vi "TEST Object Manual Bounds (Splitter).vi"() -> ()   [LabVIEW 2021, in "IObject.lvclass"]
uses:
  IObject.lvclass
  <vilib>/Utility/miscctls.llb/LVRectTypeDef.ctl
  Object/Object.lvclass
  C:/Projects/Dynamic-Scaling/Dynamic Scaling/IObject.lvclass
  IContainer/Viewport/Viewport.lvclass
  IContainer/Divider/Divider.lvclass
panel:
  in  "Vertical? [F, hor.]":bool=TRUE
  in  "OK Button 4":bool
  in  "OK Button 3":dbl(graph)
  in  "OK Button 2":dbl(graph)
  in  "Bounds":T1={"Left"=200, "Top"=20, "Right"=550, "Bottom"=190}
  in  "OK Button 1":bool
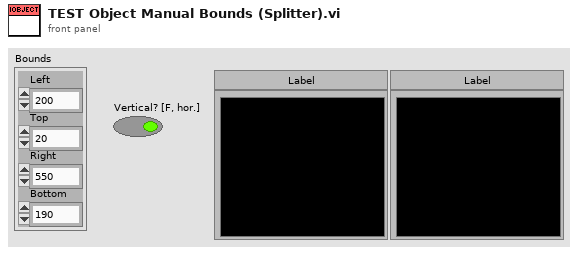
[diagram p1: front panel]
types:
  T1 = typedef "LVRectTypeDef.ctl" = cluster{"Left":i16, "Top":i16, "Right":i16, "Bottom":i16}
  T2 = cluster{"Left":dbl, "Top":dbl, "Right":dbl, "Bottom":dbl}[]
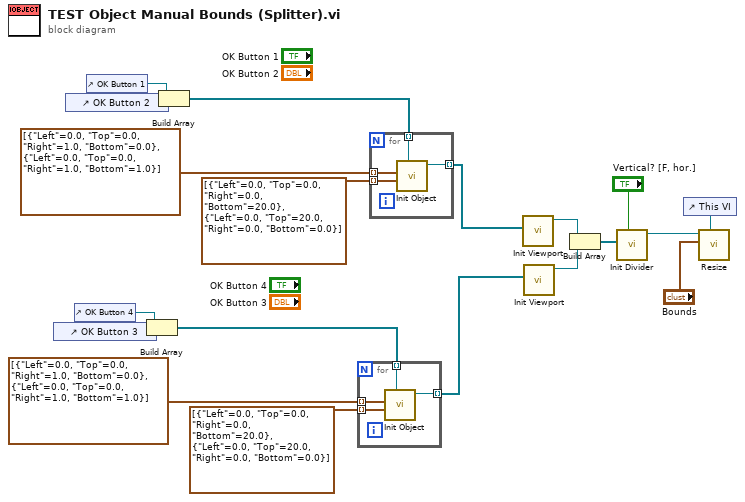
[diagram p0: block diagram]
diagram:
  n1 = control-ref of="OK Button 3"() -> (w7:refnum<vi>)
  n2 = control-ref of="OK Button 2"() -> (w18:refnum<vi>)
  n3 = control-ref of="OK Button 4"() -> (w6:refnum<vi>)
  n4 = control-ref of="OK Button 1"() -> (w19:refnum<vi>)
  n5 = Build Array(w6, w7) -> (w8:refnum<vi>[])
  n6 = Build Array(w19, w18) -> (w17:refnum<vi>[])
  n7 = for {
    tunnel: T2 [{"Left"=0.0, "Top"=0.0, "Right"=1.0, "Bottom"=0.0}, {"Left"=0.0, "Top"=0.0, "Right"=1.0, "Bottom"=1.0}] -> [w23] mode=indexing
    tunnel: w8 -> [w22] mode=indexing
    tunnel: T2 [{"Left"=0.0, "Top"=0.0, "Right"=0.0, "Bottom"=20.0}, {"Left"=0.0, "Top"=20.0, "Right"=0.0, "Bottom"=0.0}] -> [w21] mode=indexing
    tunnel: [w20] -> w11 mode=indexing
    n8 = call "Init Object.vi"("GObj Refnum"=w22, "B [0, 0, 0, 0]"=w21, "A [0, 0, 1, 1]"=w23) -> ("MMI Scaling out"=w20:refnum<class "Object.lvclass">)  [unwired: 7 in, 1 out]
  }
  n9 = for {
    tunnel: T2 [{"Left"=0.0, "Top"=0.0, "Right"=1.0, "Bottom"=0.0}, {"Left"=0.0, "Top"=0.0, "Right"=1.0, "Bottom"=1.0}] -> [w27] mode=indexing
    tunnel: w17 -> [w26] mode=indexing
    tunnel: T2 [{"Left"=0.0, "Top"=0.0, "Right"=0.0, "Bottom"=20.0}, {"Left"=0.0, "Top"=20.0, "Right"=0.0, "Bottom"=0.0}] -> [w25] mode=indexing
    tunnel: [w24] -> w13 mode=indexing
    n10 = call "Init Object.vi"("GObj Refnum"=w26, "B [0, 0, 0, 0]"=w25, "A [0, 0, 1, 1]"=w27) -> ("MMI Scaling out"=w24:refnum<class "Object.lvclass">)  [unwired: 7 in, 1 out]
  }
  n11 = call "Init Viewport.vi"("Items"=w13) -> ("Viewport out"=w5:refnum<class "Viewport.lvclass">)  [unwired: 9 in, 1 out]
  n12 = call "Init Viewport.vi"("Items"=w11) -> ("Viewport out"=w4:refnum<class "Viewport.lvclass">)  [unwired: 9 in, 1 out]
  n13 = Build Array(w5, w4) -> (w3:refnum<class "Viewport.lvclass">[])
  n14 = call "Init Divider.vi"("Vertical? [F, hor.]"="Vertical? [F, hor.]", "Items"=w3) -> ("Divider out"=w2:refnum<class "Divider.lvclass">)  [unwired: 8 in, 1 out]
  n15 = control-ref of="This VI"() -> (w14:refnum<vi>)
  n16 = call-dynamic "Resize.vi"("VI Refnum"=w14, "Bounds"="Bounds", "MMI Scaling in"=w2) -> ()  [unwired: 6 in, 3 out]
